vi "Transmit.vi"(8 "error in (no error)":errorcluster, 9 "timeout in ms (-1)":i32=-1, 10 "Packet Data":u8[](array[numeric]), 11 "Network_Streams in":T1) -> (0 "error out":errorcluster, 1 "Timeout?":bool, 2 "Packet Data Sent":u8[](array[numeric]), 3 "Network_Streams out":T1)   [LabVIEW 2020, in "Communication VIs.lvlib" / "Network.lvlib"]
uses:
  Network.lvlib
  Network Streams.ctl
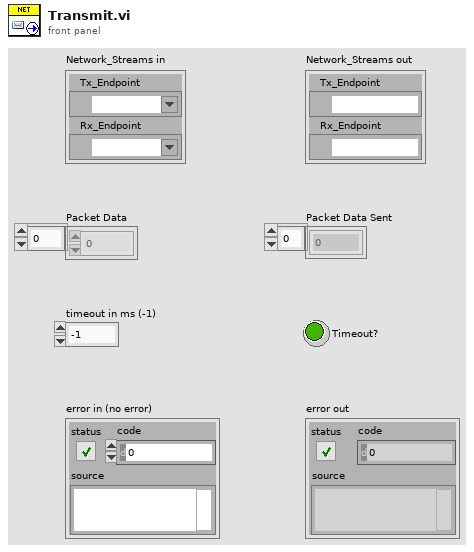
[diagram p1: front panel]
types:
  T1 = typedef "Communication VIs.lvlib/Network.lvlib/Network Streams.ctl" = cluster{"Tx_Endpoint":refnum<k21>, "Rx_Endpoint":refnum<k21>}
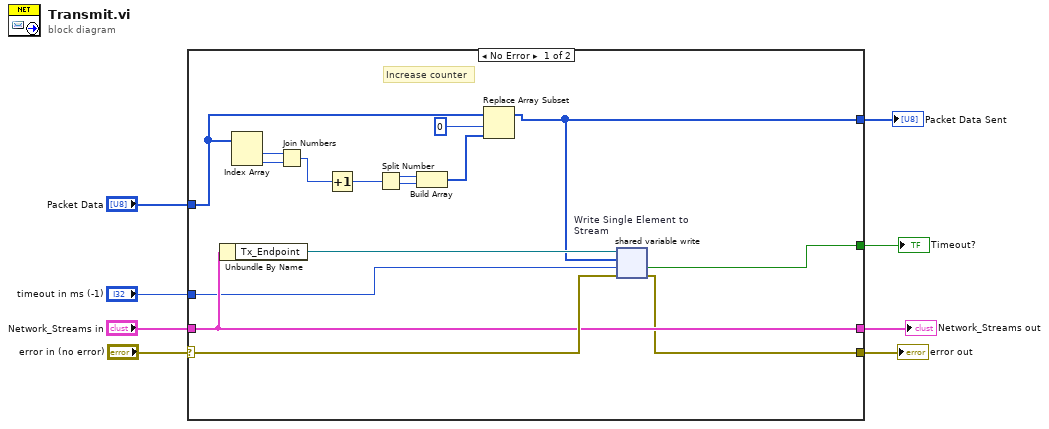
[diagram p0: block diagram]
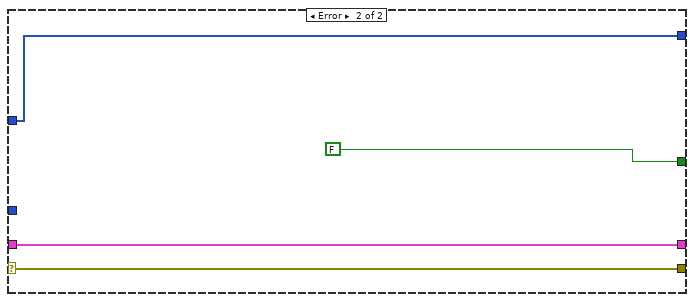
[diagram p2: hidden frame]
diagram:
  n1 = case shown="No Error" "error in (no error)" {
    selector: "error in (no error)" -> [w24 w27]
    tunnel: "timeout in ms (-1)" -> [w19 _]
    tunnel: [w20 w27] -> w5
    tunnel: [w21 FALSE ("timed out?")] -> w6
    tunnel: "Network_Streams in" -> [w23 w26]
    tunnel: [w23 w26] -> w2
    tunnel: "Packet Data" -> [w13 w25]
    tunnel: [w9 w25] -> w1
    frame No Error {
      # "Increase counter"
      n2 = Unbundle By Name(w23) -> ("Tx_Endpoint"=w22:refnum<k21>)
      n3 = Index Array(array=w13) -> (element #1=w12:u8, element #2=w11:u8)  [unwired: 2 in]
      n4 = Join Numbers(hi=w12, lo=w11) -> ((hi.lo)=w10:u16)
      n5 = Increment(x=w10) -> (x+1=w14:u16)
      n6 = Split Number(x=w14) -> (hi(x)=w18:u8, lo(x)=w17:u8)
      n7 = Build Array(w18, w17) -> (w16:u8[])
      n8 = Replace Array Subset "Replace Array Subset"(array=w13, new element=w16, index=0) -> (w9:u8[])
      n9 = shared-variable-write "Write Single Element to Stream"(w22, w24, w9, w19) -> (w20:errorcluster, w21:bool)  [unwired: 1 out]
    }
    frame Error {
    }
  }
  "error out" <- w5
  "Timeout?" <- w6
  "Network_Streams out" <- w2
  "Packet Data Sent" <- w1
